vi "Comparison of Streaming File Formats.vi"() -> ()   [LabVIEW 2023]
doc: "The Comparison of Streaming File Formats example acquires images and then saves them to disk using a variety of file formats and options. Then it reads those images from disk and compares them with the original acquired images to report the file size, write time, and whether the saved image exactly matches the acquired image. \n\nIt's important to note this example only saves a few images and you may see different results when saving a larger number of images. You should also ensure the drive where the files are saved matches the desired location since different drives may have different performance. \n\nTo view an example of how to acquire images from a camera while saving to disk, see the Stream to Disk examples."
uses:
  <vilib>/Utility/miscctls.llb/LVRowAndColumnUnsignedTypeDef.ctl
  <vilib>/vision/Avi.llb/IMAQ AVI2 Codec Path.ctl
  <vilib>/Analysis/baseanly.llb/Mean (DBL).vi
  <vilib>/Utility/High Resolution Relative Seconds.vi
  SubVIs/TDMS File Initialization (Write).vi
  <vilib>/vision/EDVR.llb/IMAQ ImageToEDVR.vi
  <vilib>/vision/EDVR.llb/IMAQ ImageToEDVR 1D U8.vi
  <vilib>/vision/EDVR.llb/IMAQ ImageToEDVR 1D I16.vi
  <vilib>/vision/EDVR.llb/IMAQ ImageToEDVR 1D U32.vi
  <vilib>/vision/EDVR.llb/IMAQ ImageToEDVR 1D U16.vi
  SubVIs/TDMS File Initialization (Read).vi
  <vilib>/Analysis/NI_AALBase.lvlib
  <vilib>/vision/driver/NI_Vision_Acquisition_Software.lvlib
panel:
  out "TDMS Disable Buffering":bool
  in  "Number of Images to Save for Each File Format":u32=25
  in  "Show Only Lossless":bool=TRUE
  out "Destination Folder":path
  in  "Camera Name":refnum<k21> caption="IMAQdx Session"
  in  "Stop":bool
  in  "Sort By":enum16{"Write Time", "File Size"}(ring)
  out "Results":i32(listbox)=-1
  out "Progress Bar":i32(slide) max=39 scale=0.0..39.0
  # "Overview: Demonstrates how to save images to disk using a variety of file formats and then reads them back and compares file size, write time, and whether the saved image exactly maches the acquired image. \nRequirements: Vision Acquisition Software.\nInstructions:\n1. Select the Camera Name.\n2. Run the VI\n3. When the table is populated, use Show Only Lossless and Sort By to modify the displayed results."
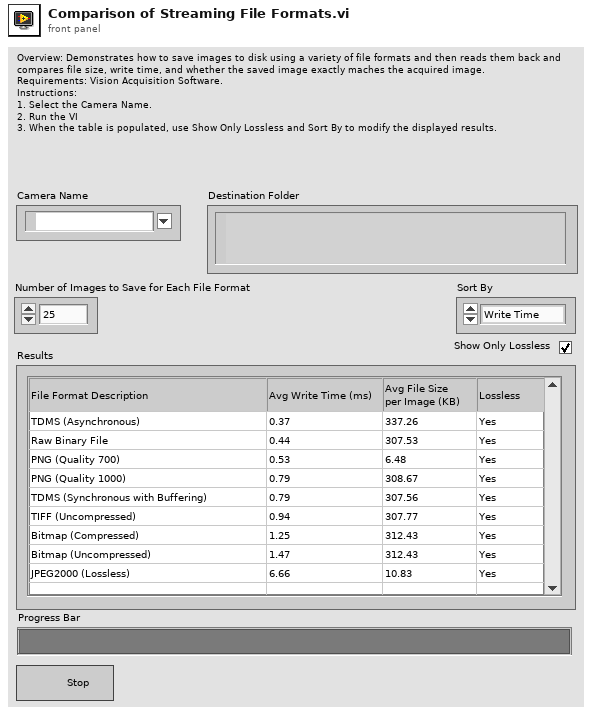
[diagram p1: front panel]
types:
  T1 = typedef "LVRowAndColumnUnsignedTypeDef.ctl" = cluster{"Row":u32, "Column":u32}
  T2 = enum8{"Enabled", "Disabled", "Disabled and Grayed Out"}
  T3 = typedef "IMAQ Image.ctl" = refnum<image>
  T4 = typedef "IMAQdx.ctl" = refnum<k21>
  T5 = typedef "Image Type" = u32
  T6 = cluster{"Rows Per Strip":i32, "Photometric":i32, "Compression Type":i32}
  T7 = cluster{"Asynchronous":bool, "Disable Buffering if Supported":bool, "Reserved Images":i64, "Fail if Reservation Fails":bool}
  T8 = enum16{"open", "replace", "create", "open or create", "replace or create", "replace or create with confirmation"}
  T9 = cluster{"Table Data":string[], "Description":string, "Write time":dbl, "File Size":dbl, "Sort Quality":dbl}
  T10 = typedef "IMAQ AVI2 Codec Path.ctl" = u32
  T11 = cluster{"Image Type":T5, "Async File Format":bool}
  T12 = cluster{"Asynchronous Write":bool, "Reserve Disk Space":bool, "Disable Buffering":bool}
  T13 = typedef "IMAQ AVI2 Refnum.ctl" = refnum<k20>
  T14 = typedef "TDMS Read Data.ctl" = cluster{"Image Type":T5, "Width":u32, "Height":u32, "Pixels per Image":u32, "Total Width":u32, "Left Offset":u32, "Image":T3}
  T15 = cluster{"Write time":dbl, "Sort Quality":dbl, "Table Data":string[]}
  T16 = cluster{"Write time":dbl, "Sort Quality":dbl, "Table Data":string[]}[]
  T17 = cluster{"File Size":dbl, "Sort Quality":dbl, "Table Data":string[]}
  T18 = cluster{"File Size":dbl, "Sort Quality":dbl, "Table Data":string[]}[]
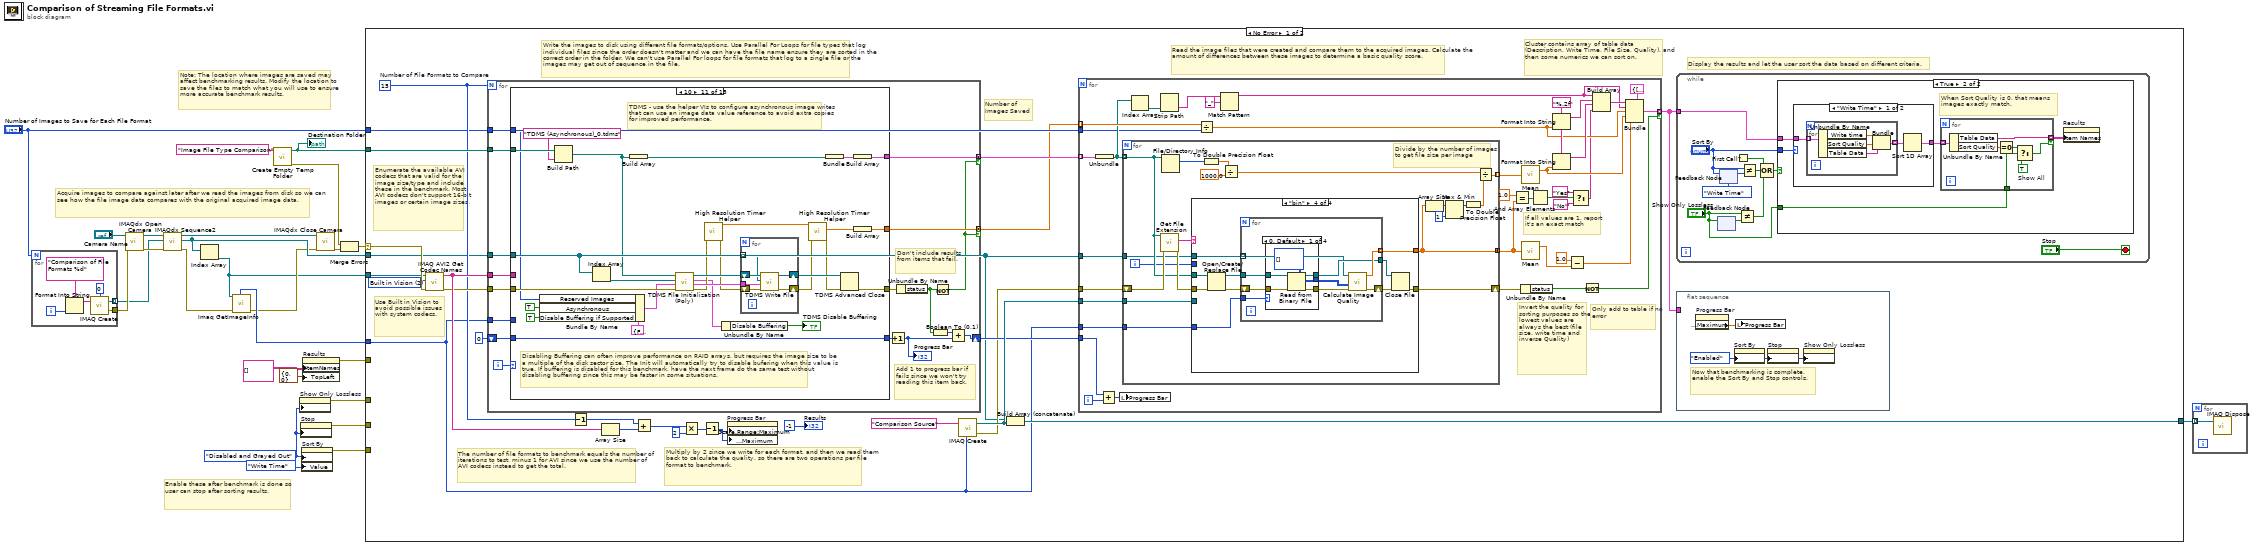
[diagram p0: block diagram]
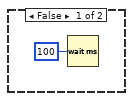
[diagram p2: hidden frame]
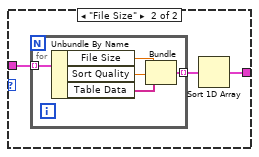
[diagram p3: hidden frame]
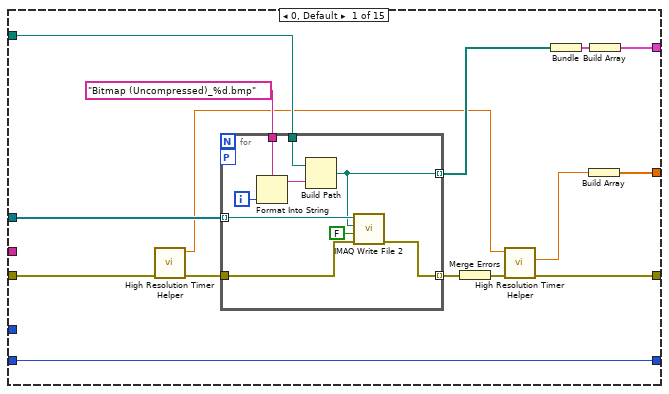
[diagram p4: hidden frame]
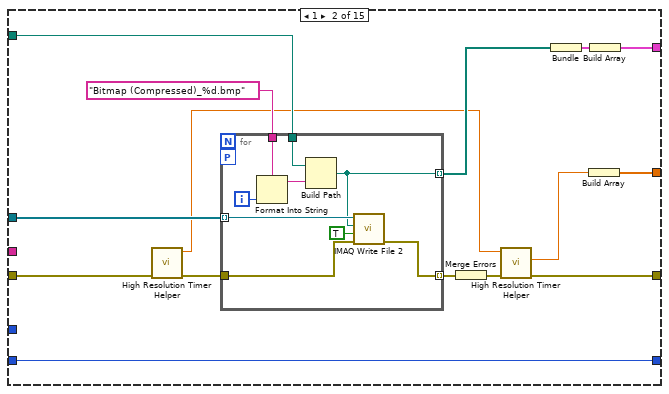
[diagram p5: hidden frame]
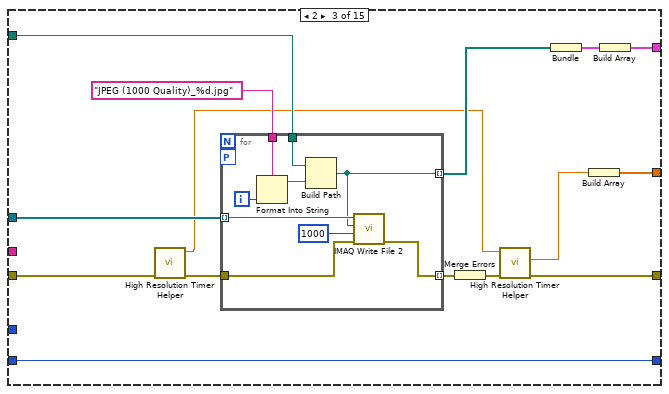
[diagram p6: hidden frame]
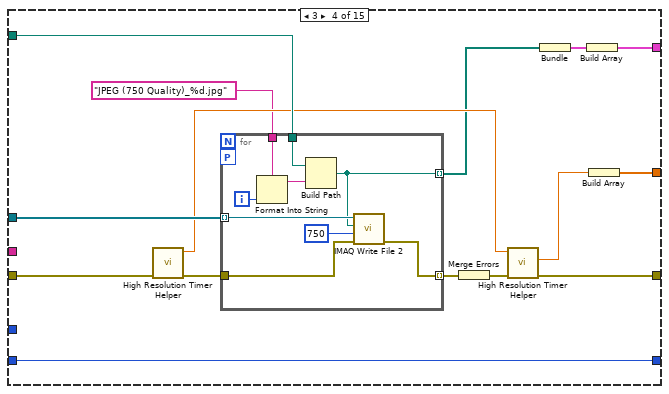
[diagram p7: hidden frame]
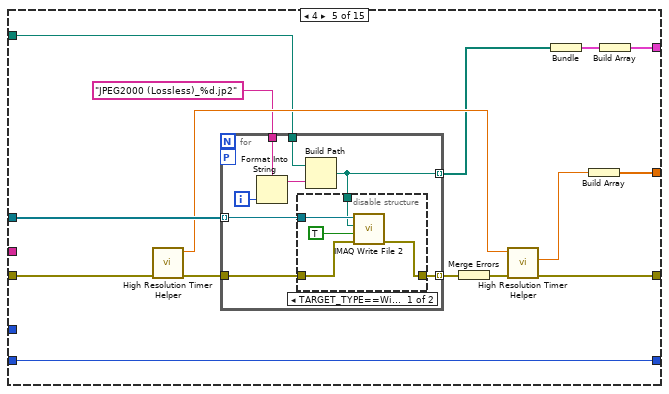
[diagram p8: hidden frame]
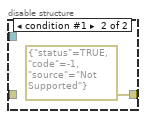
[diagram p9: hidden frame]
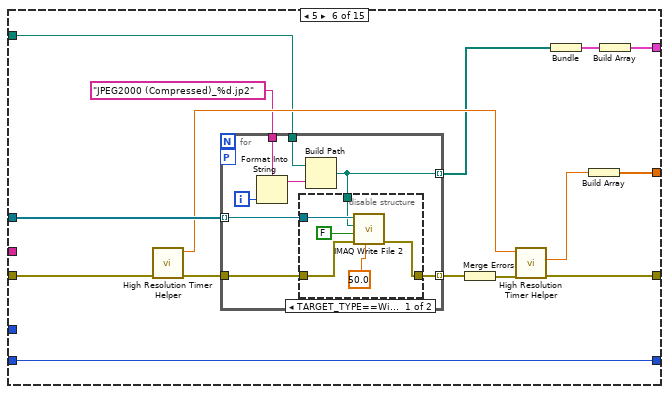
[diagram p10: hidden frame]
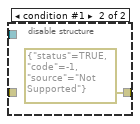
[diagram p11: hidden frame]
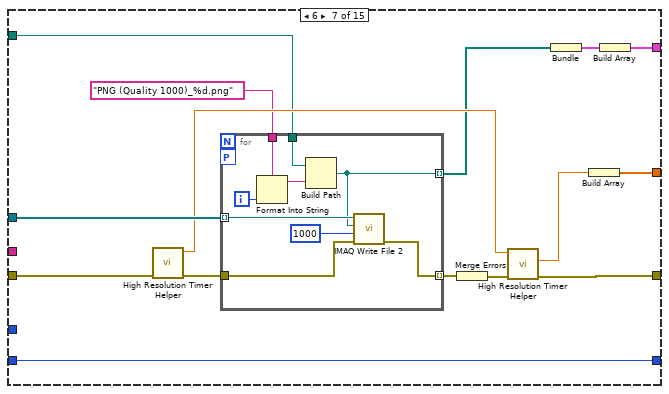
[diagram p12: hidden frame]
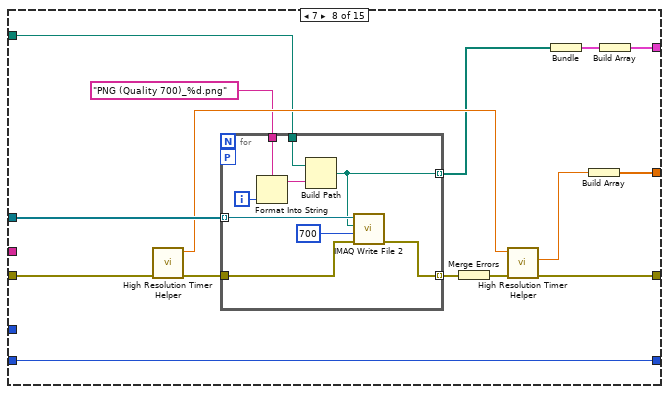
[diagram p13: hidden frame]
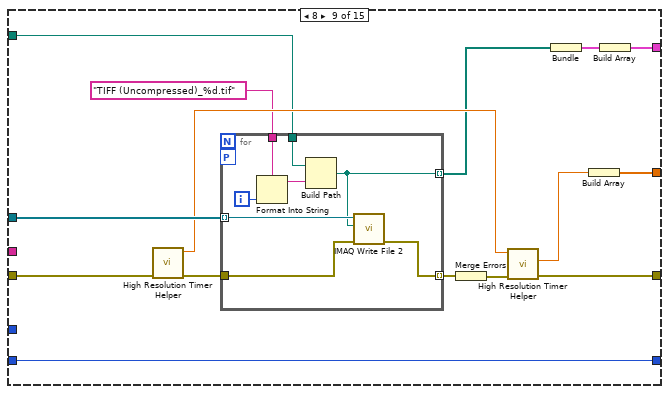
[diagram p14: hidden frame]
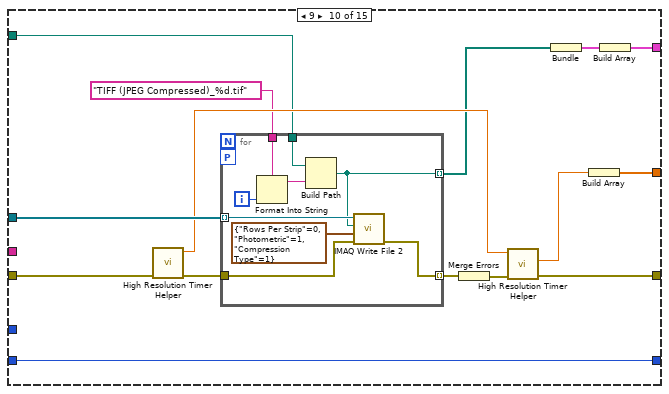
[diagram p15: hidden frame]
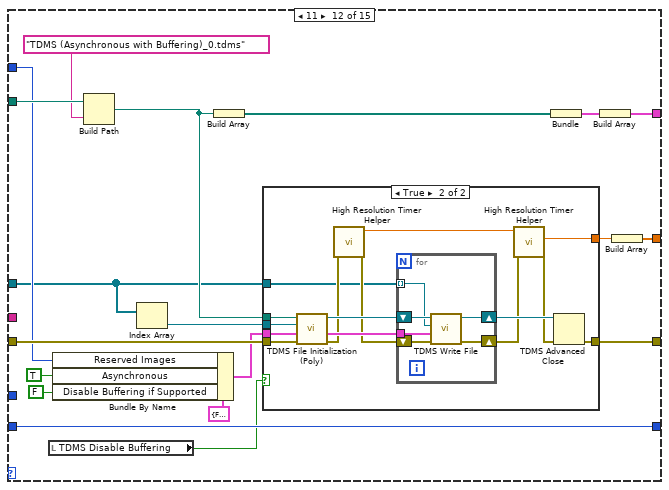
[diagram p16: hidden frame]
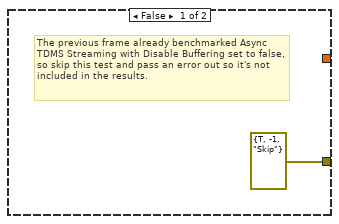
[diagram p17: hidden frame]
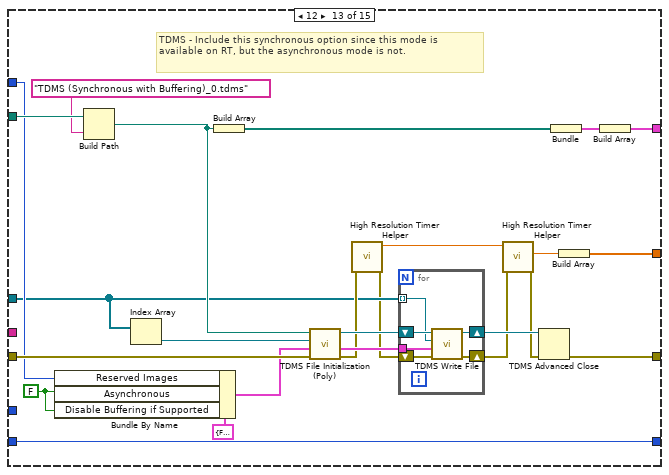
[diagram p18: hidden frame]
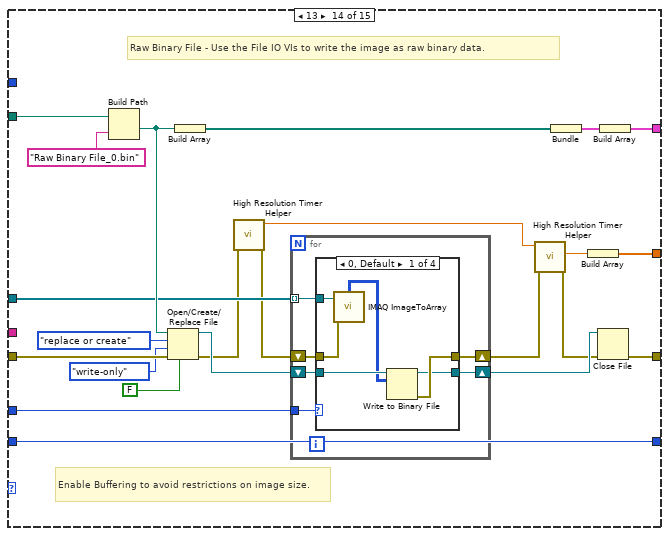
[diagram p19: hidden frame]
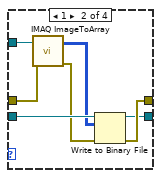
[diagram p20: hidden frame]
diagram:
  w16 = T2."Disabled and Grayed Out" ("Disabled")
  # "Note: The location where images are saved may affect benchmarking results. Modify the location to save the files to match what you will use to ensure more accurate benchmark results."
  # "Enable these after benchmark is done so user can stop after sorting results."
  # "Acquire images to compare against later after we read the images from disk so we can see how the file image data compares with the original acquired image data."
  n1 = for {
    N: "Number of Images to Save for Each File Format" -> [_]
    tunnel: [w32] -> w10
    tunnel: [w28] -> w1 mode=indexing
    i -> [w29]
    n2 = Format Into String(format string="Comparison of File Formats %d", w29) -> (resulting string=w30:string)  [unwired: 2 in, 1 out]
    n3 = call "IMAQ Create"("Border Size"=0, "Image Name"=w30) -> ("New Image"=w28:T3, "error out"=w32:errorcluster)  [unwired: 3 in]
  }
  n4 = call <vilib>:"IMAQdx Open Camera.vi"("error in"=w10, "Session In"="Camera Name") -> ("error out"=w8:errorcluster, "Session Out"=w9:T4)  [unwired: 8 in]
  n5 = call <vilib>:"IMAQdx Sequence2.vi"("error in"=w8, "Images In"=w1, "Session In"=w9) -> ("error out"=w7:errorcluster, "Images Out"=w5:T3[], "Session Out"=w6:T4)  [unwired: 6 in]
  n6 = Index Array(array=w5) -> (element=w2:T3)  [unwired: 1 in]
  n7 = call "Imaq GetImageInfo"("error in (no error)"=w7, "Image"=w2) -> ("error out"=w4:errorcluster, "Image Type"=w11:T5)  [unwired: 2 in, 6 out]
  n8 = call "Create Empty Temp Folder.vi"("Folder Name"="Image File Type Comparison") -> ("error out"=w12:errorcluster, "Empty Temp Folder"=w13:path)  [unwired: 9 in]
  "Destination Folder" <- w13
  n9 = property on="Show Only Lossless" class="Bool (strict)"("DisabledEnum"=w16) -> (error out=w15:errorcluster)  [unwired: 2 in, 1 out]
  n10 = property on="Stop" class="Bool"("DisabledEnum"=w16) -> (error out=w25:errorcluster)  [unwired: 2 in, 1 out]
  n11 = property on="Sort By" class="Enum (strict)"("DisabledEnum"=w16, "Value"=enum16{"Write Time", "File Size"}."Write Time" ("Sort By")) -> (error out=w24:errorcluster)  [unwired: 2 in, 1 out]
  n12 = property on="Results" class="MCListbox (strict)"("ItemNames"=string[][] [] ("Item Names"), "TopLeft"=T1 {"Row"=0, "Column"=0} ("Top Left Visible Cell")) -> (error out=w19:errorcluster)  [unwired: 2 in, 1 out]
  n13 = call <vilib>:"IMAQdx Close Camera.vi"("error in"=w4, "Session In"=w6) -> ("error out"=w22:errorcluster)  [unwired: 9 in]
  n14 = Merge Errors(w12, w22) -> (w21:errorcluster)
  n15 = case shown="No Error" w21 {
    selector: w21 -> [w42 w718]
    tunnel: [w54 w717] -> w26
    tunnel: w13 -> [w52 _]
    tunnel: w5 -> [w35 w717]
    tunnel: w25 -> [_ _]
    tunnel: w24 -> [_ _]
    tunnel: w19 -> [_ _]
    tunnel: w15 -> [_ _]
    tunnel: w11 -> [w38 _]
    tunnel: "Number of Images to Save for Each File Format" -> [w36 _]
    tunnel: w2 -> [w37 _]
    frame No Error {
      w34 = T10 2 items=["Default", "System", "Built in Vision"] ("Codec Source")
      w44 = 15  # Number of File Formats to Compare
      # "Use Built in Vision to avoid possible issues with system codecs."
      # "Number of Images Saved"
      # "Cluster contains array of table data (Description, Write Time, File Size, Quality), and then some numerics we can sort on."
      # "Display the results and let the user sort the data based on different criteria."
      # "The number of file formats to benchmark equals the number of iterations to test, minus 1 for AVI since we use the number of AVI codecs instead to get the total."
      # "Write the images to disk using different file formats/options. Use Parallel For Loops for file types that log individual files since the order doesn't matter and we can have the file name ensure they are sorted in the correct order in the folder. We can't use Parallel For loops for file formats that log to a single file or the images may get out of sequence in the file."
      # "Read the image files that were created and compare them to the acquired images. Calculate the amount of differences between these images to determine a basic quality score."
      # "Multiply by 2 since we write for each format, and then we read them back to calculate the quality, so there are two operations per file format to benchmark."
      # "Enumerate the available AVI codecs that are valid for the image size/type and include these in the benchmark. Most AVI codecs don't support 16-bit images or certain image sizes."
      n16 = call "IMAQ AVI2 Get Codec Names"("error in (no error)"=w42, "Codec Source"=w34, "Image"=w37) -> ("error out"=w48:errorcluster, "Codec Names"=w51:string[])  [unwired: 7 out]
      n17 = for {
        N: w44 -> [_]
        tunnel: [w117] -> w33 mode=concatenating if=w109
        tunnel: w52 -> [w116]
        tunnel: w51 -> [w115]
        tunnel: w48 -> [w114]
        tunnel: w35 -> [w113]
        tunnel: [w112] -> w46 mode=concatenating if=w109
        shift-right: [w106] -> w45
        shift-left: 0 -> [w111]
        tunnel: w38 -> [w110]
        tunnel: w36 -> [w101]
        i -> [w102]
        # "Add 1 to progress bar if fails since we won't try reading this item back."
        # "Don't include results from items that fail."
        n18 = case shown="10" w102 {
          tunnel: [w131 w155 w179 w202 w225 w254 w284 w308 w332 w355 w395 w420 w467 w496 w537] -> w117
          tunnel: [w120 w144 w168 w198 w218 w247 w277 w301 w325 w348 w386 w411 w460 w484 w536] -> w103
          tunnel: w116 -> [w130 w154 w178 w201 w224 w253 w283 w307 w331 w354 w390 w415 w463 w492 w535]
          tunnel: w115 -> [_ _ _ _ _ _ _ _ _ _ _ _ _ _ w534]
          tunnel: w114 -> [w123 w147 w171 w203 w226 w255 w285 w309 w333 w356 w391 w416 w456 w488 w533]
          tunnel: w113 -> [w132 w156 w180 w204 w228 w257 w287 w311 w335 w358 w370 w403 w445 w480 w531]
          tunnel: [w129 w153 w177 w200 w220 w249 w279 w303 w327 w350 w393 w418 w465 w494 w532] -> w112
          tunnel: w111 -> [w125 w149 w176 w199 w219 w248 w278 w302 w326 w349 w392 w417 w464 w493 w530]
          tunnel: [w125 w149 w176 w199 w219 w248 w278 w302 w326 w349 w392 w417 w464 w493 w529] -> w105
          tunnel: w110 -> [_ _ _ _ _ _ _ _ _ _ _ _ _ w489 _]
          tunnel: w101 -> [_ _ _ _ _ _ _ _ _ _ w368 w404 w446 _ _]
          frame 0, Default {
            n19 = call "High Resolution Timer Helper.vi"("error in (no error)"=w123) -> ("error out"=w122:errorcluster, "Current Time"=w119:dbl)  [unwired: 8 in, 1 out]
            n20 = for {
              tunnel: w132 -> [w141] mode=indexing
              tunnel: w130 -> [w139]
              tunnel: "Bitmap (Uncompressed)_%d.bmp" -> [w137]
              tunnel: [w135] -> w127 mode=indexing
              workers-P: _ -> [_]
              tunnel: w122 -> [w134]
              tunnel: [w133] -> w124 mode=indexing
              i -> [w138]
              n21 = Format Into String(format string=w137, w138) -> (resulting string=w136:string)  [unwired: 2 in, 1 out]
              n22 = Build Path(base path=w139, name or relative path=w136) -> (appended path=w135:path)
              n23 = call-poly "IMAQ Write File 2"("error in (no error)"=w134, "Compress? (N)"=FALSE, "File Path"=w135, "Image"=w141) -> ("error out"=w133:errorcluster)  [unwired: 6 in, 1 out]
            }
            n24 = Merge Errors(w124) -> (w121:errorcluster)
            n25 = call "High Resolution Timer Helper.vi"("error in (no error)"=w121, "Previous Time"=w119) -> ("error out"=w120:errorcluster, "Time Difference (ms)"=w118:dbl)  [unwired: 7 in, 1 out]
            n26 = Bundle(w127) -> (w126:cluster{path[]})  [unwired: 1 in]
            n27 = Build Array(w118) -> (w131:dbl[])
            n28 = Build Array(w126) -> (w129:cluster{path[]}[])
          }
          frame 1 {
            n29 = call "High Resolution Timer Helper.vi"("error in (no error)"=w147) -> ("error out"=w146:errorcluster, "Current Time"=w142:dbl)  [unwired: 8 in, 1 out]
            n30 = for {
              tunnel: w156 -> [w165] mode=indexing
              tunnel: w154 -> [w163]
              tunnel: "Bitmap (Compressed)_%d.bmp" -> [w161]
              tunnel: [w159] -> w151 mode=indexing
              workers-P: _ -> [_]
              tunnel: w146 -> [w158]
              tunnel: [w157] -> w148 mode=indexing
              i -> [w162]
              n31 = Format Into String(format string=w161, w162) -> (resulting string=w160:string)  [unwired: 2 in, 1 out]
              n32 = Build Path(base path=w163, name or relative path=w160) -> (appended path=w159:path)
              n33 = call-poly "IMAQ Write File 2"("error in (no error)"=w158, "Compress? (N)"=TRUE, "File Path"=w159, "Image"=w165) -> ("error out"=w157:errorcluster)  [unwired: 6 in, 1 out]
            }
            n34 = Merge Errors(w148) -> (w145:errorcluster)
            n35 = call "High Resolution Timer Helper.vi"("error in (no error)"=w145, "Previous Time"=w142) -> ("error out"=w144:errorcluster, "Time Difference (ms)"=w143:dbl)  [unwired: 7 in, 1 out]
            n36 = Bundle(w151) -> (w150:cluster{path[]})  [unwired: 1 in]
            n37 = Build Array(w143) -> (w155:dbl[])
            n38 = Build Array(w150) -> (w153:cluster{path[]}[])
          }
          frame 2 {
            n39 = call "High Resolution Timer Helper.vi"("error in (no error)"=w171) -> ("error out"=w170:errorcluster, "Current Time"=w166:dbl)  [unwired: 8 in, 1 out]
            n40 = for {
              tunnel: w180 -> [w189] mode=indexing
              tunnel: w178 -> [w188]
              tunnel: "JPEG (1000 Quality)_%d.jpg" -> [w186]
              tunnel: [w184] -> w174 mode=indexing
              workers-P: _ -> [_]
              tunnel: w170 -> [w182]
              tunnel: [w181] -> w172 mode=indexing
              i -> [w187]
              n41 = Format Into String(format string=w186, w187) -> (resulting string=w185:string)  [unwired: 2 in, 1 out]
              n42 = Build Path(base path=w188, name or relative path=w185) -> (appended path=w184:path)
              n43 = call-poly "IMAQ Write File 2"("error in (no error)"=w182, "Image Quality"=u32 1000, "File Path"=w184, "Image"=w189) -> ("error out"=w181:errorcluster)  [unwired: 6 in, 1 out]
            }
            n44 = Merge Errors(w172) -> (w169:errorcluster)
            n45 = call "High Resolution Timer Helper.vi"("error in (no error)"=w169, "Previous Time"=w166) -> ("error out"=w168:errorcluster, "Time Difference (ms)"=w167:dbl)  [unwired: 7 in, 1 out]
            n46 = Bundle(w174) -> (w173:cluster{path[]})  [unwired: 1 in]
            n47 = Build Array(w167) -> (w179:dbl[])
            n48 = Build Array(w173) -> (w177:cluster{path[]}[])
          }
          frame 3 {
            n49 = call "High Resolution Timer Helper.vi"("error in (no error)"=w203) -> ("error out"=w192:errorcluster, "Current Time"=w197:dbl)  [unwired: 8 in, 1 out]
            n50 = for {
              tunnel: w204 -> [w213] mode=indexing
              tunnel: w201 -> [w212]
              tunnel: "JPEG (750 Quality)_%d.jpg" -> [w210]
              tunnel: [w208] -> w195 mode=indexing
              workers-P: _ -> [_]
              tunnel: w192 -> [w206]
              tunnel: [w205] -> w191 mode=indexing
              i -> [w211]
              n51 = Format Into String(format string=w210, w211) -> (resulting string=w209:string)  [unwired: 2 in, 1 out]
              n52 = Build Path(base path=w212, name or relative path=w209) -> (appended path=w208:path)
              n53 = call-poly "IMAQ Write File 2"("error in (no error)"=w206, "Image Quality"=u32 750, "File Path"=w208, "Image"=w213) -> ("error out"=w205:errorcluster)  [unwired: 6 in, 1 out]
            }
            n54 = Merge Errors(w191) -> (w190:errorcluster)
            n55 = call "High Resolution Timer Helper.vi"("error in (no error)"=w190, "Previous Time"=w197) -> ("error out"=w198:errorcluster, "Time Difference (ms)"=w193:dbl)  [unwired: 7 in, 1 out]
            n56 = Bundle(w195) -> (w194:cluster{path[]})  [unwired: 1 in]
            n57 = Build Array(w194) -> (w200:cluster{path[]}[])
            n58 = Build Array(w193) -> (w202:dbl[])
          }
          frame 4 {
            n59 = call "High Resolution Timer Helper.vi"("error in (no error)"=w226) -> ("error out"=w216:errorcluster, "Current Time"=w227:dbl)  [unwired: 8 in, 1 out]
            n60 = for {
              tunnel: w228 -> [w236] mode=indexing
              tunnel: w224 -> [w235]
              tunnel: "JPEG2000 (Lossless)_%d.jp2" -> [w233]
              tunnel: [w231] -> w222 mode=indexing
              workers-P: _ -> [_]
              tunnel: w216 -> [w230]
              tunnel: [w229] -> w215 mode=indexing
              i -> [w234]
              n61 = Format Into String(format string=w233, w234) -> (resulting string=w232:string)  [unwired: 2 in, 1 out]
              n62 = Build Path(base path=w235, name or relative path=w232) -> (appended path=w231:path)
              n63 = disable-structure shown="TARGET_TYPE==Windows" {
                disable-tunnel: w236 -> [w241 _]
                disable-tunnel: w230 -> [w240 _]
                disable-tunnel: [w239 errorcluster {"status"=TRUE, "code"=-1, "source"="Not Supported"} ("error out")] -> w229
                disable-tunnel: w231 -> [w238 _]
                frame condition #0 (active) {
                  n64 = call-poly "IMAQ Write File 2"("error in (no error)"=w240, "Lossless? (true)"=TRUE, "File Path"=w238, "Image"=w241) -> ("error out"=w239:errorcluster)  [unwired: 6 in, 1 out]
                }
                frame condition #1 {
                }
              }
            }
            n65 = Merge Errors(w215) -> (w214:errorcluster)
            n66 = call "High Resolution Timer Helper.vi"("error in (no error)"=w214, "Previous Time"=w227) -> ("error out"=w218:errorcluster, "Time Difference (ms)"=w217:dbl)  [unwired: 7 in, 1 out]
            n67 = Bundle(w222) -> (w221:cluster{path[]})  [unwired: 1 in]
            n68 = Build Array(w217) -> (w225:dbl[])
            n69 = Build Array(w221) -> (w220:cluster{path[]}[])
          }
          frame 5 {
            n70 = call "High Resolution Timer Helper.vi"("error in (no error)"=w255) -> ("error out"=w245:errorcluster, "Current Time"=w256:dbl)  [unwired: 8 in, 1 out]
            n71 = for {
              tunnel: w257 -> [w265] mode=indexing
              tunnel: w253 -> [w264]
              tunnel: "JPEG2000 (Compressed)_%d.jp2" -> [w262]
              tunnel: [w260] -> w251 mode=indexing
              workers-P: _ -> [_]
              tunnel: w245 -> [w259]
              tunnel: [w258] -> w244 mode=indexing
              i -> [w263]
              n72 = Format Into String(format string=w262, w263) -> (resulting string=w261:string)  [unwired: 2 in, 1 out]
              n73 = Build Path(base path=w264, name or relative path=w261) -> (appended path=w260:path)
              n74 = disable-structure shown="TARGET_TYPE==Windows" {
                disable-tunnel: w265 -> [w271 _]
                disable-tunnel: w259 -> [w270 _]
                disable-tunnel: [w269 errorcluster {"status"=TRUE, "code"=-1, "source"="Not Supported"} ("error out")] -> w258
                disable-tunnel: w260 -> [w268 _]
                frame condition #0 (active) {
                  n75 = call-poly "IMAQ Write File 2"("Compression Ratio"=sgl 50.0, "error in (no error)"=w270, "Lossless? (true)"=FALSE, "File Path"=w268, "Image"=w271) -> ("error out"=w269:errorcluster)  [unwired: 5 in, 1 out]
                }
                frame condition #1 {
                }
              }
            }
            n76 = Merge Errors(w244) -> (w243:errorcluster)
            n77 = call "High Resolution Timer Helper.vi"("error in (no error)"=w243, "Previous Time"=w256) -> ("error out"=w247:errorcluster, "Time Difference (ms)"=w246:dbl)  [unwired: 7 in, 1 out]
            n78 = Bundle(w251) -> (w250:cluster{path[]})  [unwired: 1 in]
            n79 = Build Array(w246) -> (w254:dbl[])
            n80 = Build Array(w250) -> (w249:cluster{path[]}[])
          }
          frame 6 {
            n81 = call "High Resolution Timer Helper.vi"("error in (no error)"=w285) -> ("error out"=w275:errorcluster, "Current Time"=w286:dbl)  [unwired: 8 in, 1 out]
            n82 = for {
              tunnel: w287 -> [w296] mode=indexing
              tunnel: w283 -> [w295]
              tunnel: "PNG (Quality 1000)_%d.png" -> [w293]
              tunnel: [w291] -> w281 mode=indexing
              workers-P: _ -> [_]
              tunnel: w275 -> [w289]
              tunnel: [w288] -> w274 mode=indexing
              i -> [w294]
              n83 = Format Into String(format string=w293, w294) -> (resulting string=w292:string)  [unwired: 2 in, 1 out]
              n84 = Build Path(base path=w295, name or relative path=w292) -> (appended path=w291:path)
              n85 = call-poly "IMAQ Write File 2"("error in (no error)"=w289, "Image Quality"=u32 1000, "File Path"=w291, "Image"=w296) -> ("error out"=w288:errorcluster)  [unwired: 6 in, 1 out]
            }
            n86 = Merge Errors(w274) -> (w273:errorcluster)
            n87 = call "High Resolution Timer Helper.vi"("error in (no error)"=w273, "Previous Time"=w286) -> ("error out"=w277:errorcluster, "Time Difference (ms)"=w276:dbl)  [unwired: 7 in, 1 out]
            n88 = Bundle(w281) -> (w280:cluster{path[]})  [unwired: 1 in]
            n89 = Build Array(w276) -> (w284:dbl[])
            n90 = Build Array(w280) -> (w279:cluster{path[]}[])
          }
          frame 7 {
            n91 = call "High Resolution Timer Helper.vi"("error in (no error)"=w309) -> ("error out"=w299:errorcluster, "Current Time"=w310:dbl)  [unwired: 8 in, 1 out]
            n92 = for {
              tunnel: w311 -> [w320] mode=indexing
              tunnel: w307 -> [w319]
              tunnel: "PNG (Quality 700)_%d.png" -> [w317]
              tunnel: [w315] -> w305 mode=indexing
              workers-P: _ -> [_]
              tunnel: w299 -> [w313]
              tunnel: [w312] -> w298 mode=indexing
              i -> [w318]
              n93 = Format Into String(format string=w317, w318) -> (resulting string=w316:string)  [unwired: 2 in, 1 out]
              n94 = Build Path(base path=w319, name or relative path=w316) -> (appended path=w315:path)
              n95 = call-poly "IMAQ Write File 2"("error in (no error)"=w313, "Image Quality"=u32 700, "File Path"=w315, "Image"=w320) -> ("error out"=w312:errorcluster)  [unwired: 6 in, 1 out]
            }
            n96 = Merge Errors(w298) -> (w297:errorcluster)
            n97 = call "High Resolution Timer Helper.vi"("error in (no error)"=w297, "Previous Time"=w310) -> ("error out"=w301:errorcluster, "Time Difference (ms)"=w300:dbl)  [unwired: 7 in, 1 out]
            n98 = Bundle(w305) -> (w304:cluster{path[]})  [unwired: 1 in]
            n99 = Build Array(w300) -> (w308:dbl[])
            n100 = Build Array(w304) -> (w303:cluster{path[]}[])
          }
          frame 8 {
            n101 = call "High Resolution Timer Helper.vi"("error in (no error)"=w333) -> ("error out"=w323:errorcluster, "Current Time"=w334:dbl)  [unwired: 8 in, 1 out]
            n102 = for {
              tunnel: w335 -> [w343] mode=indexing
              tunnel: w331 -> [w342]
              tunnel: "TIFF (Uncompressed)_%d.tif" -> [w340]
              tunnel: [w338] -> w329 mode=indexing
              workers-P: _ -> [_]
              tunnel: w323 -> [w337]
              tunnel: [w336] -> w322 mode=indexing
              i -> [w341]
              n103 = Format Into String(format string=w340, w341) -> (resulting string=w339:string)  [unwired: 2 in, 1 out]
              n104 = Build Path(base path=w342, name or relative path=w339) -> (appended path=w338:path)
              n105 = call-poly "IMAQ Write File 2"("error in (no error)"=w337, "File Path"=w338, "Image"=w343) -> ("error out"=w336:errorcluster)  [unwired: 7 in, 1 out]
            }
            n106 = Merge Errors(w322) -> (w321:errorcluster)
            n107 = call "High Resolution Timer Helper.vi"("error in (no error)"=w321, "Previous Time"=w334) -> ("error out"=w325:errorcluster, "Time Difference (ms)"=w324:dbl)  [unwired: 7 in, 1 out]
            n108 = Bundle(w329) -> (w328:cluster{path[]})  [unwired: 1 in]
            n109 = Build Array(w324) -> (w332:dbl[])
            n110 = Build Array(w328) -> (w327:cluster{path[]}[])
          }
          frame 9 {
            n111 = call "High Resolution Timer Helper.vi"("error in (no error)"=w356) -> ("error out"=w346:errorcluster, "Current Time"=w357:dbl)  [unwired: 8 in, 1 out]
            n112 = for {
              tunnel: w358 -> [w367] mode=indexing
              tunnel: w354 -> [w366]
              tunnel: "TIFF (JPEG Compressed)_%d.tif" -> [w364]
              tunnel: [w362] -> w352 mode=indexing
              workers-P: _ -> [_]
              tunnel: w346 -> [w360]
              tunnel: [w359] -> w345 mode=indexing
              i -> [w365]
              n113 = Format Into String(format string=w364, w365) -> (resulting string=w363:string)  [unwired: 2 in, 1 out]
              n114 = Build Path(base path=w366, name or relative path=w363) -> (appended path=w362:path)
              n115 = call-poly "IMAQ Write File 2"("error in (no error)"=w360, "TIFF Options"=T6 {"Rows Per Strip"=0, "Photometric"=1, "Compression Type"=1}, "File Path"=w362, "Image"=w367) -> ("error out"=w359:errorcluster)  [unwired: 6 in, 1 out]
            }
            n116 = Merge Errors(w345) -> (w344:errorcluster)
            n117 = call "High Resolution Timer Helper.vi"("error in (no error)"=w344, "Previous Time"=w357) -> ("error out"=w348:errorcluster, "Time Difference (ms)"=w347:dbl)  [unwired: 7 in, 1 out]
            n118 = Bundle(w352) -> (w351:cluster{path[]})  [unwired: 1 in]
            n119 = Build Array(w347) -> (w355:dbl[])
            n120 = Build Array(w351) -> (w350:cluster{path[]}[])
          }
          frame 10 {
            # "Disabling Buffering can often improve performance on RAID arrays, but requires the image size to be a multiple of the disk sector size. The Init will automatically try to disable bufering when this value is true. If buffering is disabled for this benchmark, have the next frame do the same test without disabling buffering since this may be faster in some situations."
            # "TDMS - use the helper VIs to configure asynchronous image writes that can use an image data value reference to avoid extra copies for improved performance."
            n121 = Bundle By Name(cluster=T7 {"Asynchronous"=FALSE, "Disable Buffering if Supported"=FALSE, "Reserved Images"=1000, "Fail if Reservation Fails"=FALSE} ("Write Settings"), "Reserved Images"=w368, "Asynchronous"=TRUE, "Disable Buffering if Supported"=TRUE ("Asynchronous")) -> (w372:T7)
            n122 = Build Path(base path=w390, name or relative path="TDMS (Asynchronous)_0.tdms") -> (appended path=w388:path)
            n123 = Index Array(array=w370) -> (element=w369:T3)  [unwired: 1 in]
            n124 = Build Array(w388) -> (w387:path[])
            n125 = call-poly "TDMS File Initialization (Poly).vi"("error in (no error)"=w391, "Write Settings"=w372, "Image In"=w369, "File Path"=w388) -> ("error out"=w382:errorcluster, "Write Settings Out"=w383:T11, "Optimizations Configured"=w376:T12, "TDMS Refnum Out"=w384:refnum<k34>)  [unwired: 4 in]
            n126 = call "High Resolution Timer Helper.vi"("error in (no error)"=w382) -> ("error out"=w381:errorcluster, "Current Time"=w378:dbl)  [unwired: 8 in, 1 out]
            n127 = Unbundle By Name(w376) -> ("Disable Buffering"=→"TDMS Disable Buffering":bool)
            n128 = for {
              tunnel: w370 -> [w398] mode=indexing
              shift-right: [w396] -> w380
              shift-left: w381 -> [w401]
              shift-right: [w397] -> w385
              shift-left: w384 -> [w400]
              tunnel: w383 -> [w399]
              n129 = call "TDMS Write File.vi"("error in"=w401, "Write Settings"=w399, "Image"=w398, "TDMS Ref In"=w400) -> ("error out"=w396:errorcluster, "TDMS Ref Out"=w397:refnum<k34>)  [unwired: 6 in]
            }
            n130 = call "High Resolution Timer Helper.vi"("error in (no error)"=w380, "Previous Time"=w378) -> ("error out"=w379:errorcluster, "Time Difference (ms)"=w377:dbl)  [unwired: 7 in, 1 out]
            n131 = Bundle(w387) -> (w394:cluster{path[]})  [unwired: 1 in]
            n132 = TDMS Advanced Close(8:w379, 11:w385) -> (0:w386:errorcluster)  [unwired: 2 in, 1 out]
            n133 = Build Array(w394) -> (w393:cluster{path[]}[])
            n134 = Build Array(w377) -> (w395:dbl[])
          }
          frame 11 {
            n135 = local read "TDMS Disable Buffering"() -> (w406:bool)
            n136 = Bundle By Name(cluster=T7 {"Asynchronous"=FALSE, "Disable Buffering if Supported"=FALSE, "Reserved Images"=1000, "Fail if Reservation Fails"=FALSE} ("Write Settings"), "Reserved Images"=w404, "Asynchronous"=TRUE, "Disable Buffering if Supported"=FALSE) -> (w409:T7)
            n137 = Build Path(base path=w415, name or relative path="TDMS (Asynchronous with Buffering)_0.tdms") -> (appended path=w413:path)
            n138 = Index Array(array=w403) -> (element=w402:T3)  [unwired: 1 in]
            n139 = Build Array(w413) -> (w412:path[])
            n140 = case shown="True" w406 {
              tunnel: w416 -> [_ w436]
              tunnel: w413 -> [_ w435]
              tunnel: [errorcluster {"status"=TRUE, "code"=-1, "source"="Skip"} ("error out") w434] -> w411
              tunnel: [_ w425] -> w410
              tunnel: w403 -> [_ w424]
              tunnel: w409 -> [_ w423]
              tunnel: w402 -> [_ w422]
              frame False {
                # "The previous frame already benchmarked Async TDMS Streaming with Disable Buffering set to false, so skip this test and pass an error out so it's not included in the results."
              }
              frame True {
                n141 = call-poly "TDMS File Initialization (Poly).vi"("error in (no error)"=w436, "Write Settings"=w423, "Image In"=w422, "File Path"=w435) -> ("error out"=w430:errorcluster, "Write Settings Out"=w431:T11, "TDMS Refnum Out"=w432:refnum<k34>)  [unwired: 4 in, 1 out]
                n142 = call "High Resolution Timer Helper.vi"("error in (no error)"=w430) -> ("error out"=w429:errorcluster, "Current Time"=w426:dbl)  [unwired: 8 in, 1 out]
                n143 = for {
                  tunnel: w424 -> [w439] mode=indexing
                  shift-right: [w437] -> w428
                  shift-left: w429 -> [w442]
                  shift-right: [w438] -> w433
                  shift-left: w432 -> [w441]
                  tunnel: w431 -> [w440]
                  n144 = call "TDMS Write File.vi"("error in"=w442, "Write Settings"=w440, "Image"=w439, "TDMS Ref In"=w441) -> ("error out"=w437:errorcluster, "TDMS Ref Out"=w438:refnum<k34>)  [unwired: 6 in]
                }
                n145 = call "High Resolution Timer Helper.vi"("error in (no error)"=w428, "Previous Time"=w426) -> ("error out"=w427:errorcluster, "Time Difference (ms)"=w425:dbl)  [unwired: 7 in, 1 out]
                n146 = TDMS Advanced Close(8:w427, 11:w433) -> (0:w434:errorcluster)  [unwired: 2 in, 1 out]
              }
            }
            n147 = Bundle(w412) -> (w419:cluster{path[]})  [unwired: 1 in]
            n148 = Build Array(w419) -> (w418:cluster{path[]}[])
            n149 = Build Array(w410) -> (w420:dbl[])
          }
          frame 12 {
            w447 = FALSE ("Asynchronous")
            # "TDMS - Include this synchronous option since this mode is available on RT, but the asynchronous mode is not."
            n150 = Bundle By Name(cluster=T7 {"Asynchronous"=FALSE, "Disable Buffering if Supported"=FALSE, "Reserved Images"=1000, "Fail if Reservation Fails"=FALSE} ("Write Settings"), "Reserved Images"=w446, "Asynchronous"=w447, "Disable Buffering if Supported"=w447) -> (w455:T7)
            n151 = Build Path(base path=w463, name or relative path="TDMS (Synchronous with Buffering)_0.tdms") -> (appended path=w458:path)
            n152 = Index Array(array=w445) -> (element=w444:T3)  [unwired: 1 in]
            n153 = Build Array(w458) -> (w461:path[])
            n154 = call-poly "TDMS File Initialization (Poly).vi"("error in (no error)"=w456, "Write Settings"=w455, "Image In"=w444, "File Path"=w458) -> ("error out"=w453:errorcluster, "Write Settings Out"=w454:T11, "TDMS Refnum Out"=w457:refnum<k34>)  [unwired: 4 in, 1 out]
            n155 = call "High Resolution Timer Helper.vi"("error in (no error)"=w453) -> ("error out"=w443:errorcluster, "Current Time"=w451:dbl)  [unwired: 8 in, 1 out]
            n156 = for {
              tunnel: w445 -> [w471] mode=indexing
              shift-right: [w469] -> w450
              shift-left: w443 -> [w473]
              shift-right: [w468] -> w459
              shift-left: w457 -> [w472]
              tunnel: w454 -> [w470]
              n157 = call "TDMS Write File.vi"("error in"=w473, "Write Settings"=w470, "Image"=w471, "TDMS Ref In"=w472) -> ("error out"=w469:errorcluster, "TDMS Ref Out"=w468:refnum<k34>)  [unwired: 6 in]
            }
            n158 = call "High Resolution Timer Helper.vi"("error in (no error)"=w450, "Previous Time"=w451) -> ("error out"=w449:errorcluster, "Time Difference (ms)"=w452:dbl)  [unwired: 7 in, 1 out]
            n159 = TDMS Advanced Close(8:w449, 11:w459) -> (0:w460:errorcluster)  [unwired: 2 in, 1 out]
            n160 = Bundle(w461) -> (w466:cluster{path[]})  [unwired: 1 in]
            n161 = Build Array(w452) -> (w467:dbl[])
            n162 = Build Array(w466) -> (w465:cluster{path[]}[])
          }
          frame 13 {
            # "Raw Binary File - Use the File IO VIs to write the image as raw binary data."
            # "Enable Buffering to avoid restrictions on image size."
            n163 = Build Path(base path=w492, name or relative path="Raw Binary File_0.bin") -> (appended path=w487:path)
            n164 = Open/Create/Replace File(file path (use dialog)=w487, error in=w488, operation (0:open)=T8."replace or create", access (0:read/write)=enum16{"read/write", "read-only", "write-only"}."write-only", disable buffering (F)=FALSE) -> (refnum out=w485:refnum<file>, error out=w479:errorcluster)  [unwired: 1 in, 1 out]
            n165 = Build Array(w487) -> (w490:path[])
            n166 = call "High Resolution Timer Helper.vi"("error in (no error)"=w479) -> ("error out"=w474:errorcluster, "Current Time"=w477:dbl)  [unwired: 8 in, 1 out]
            n167 = for {
              shift-right: [w497] -> w476
              shift-left: w474 -> [w502]
              tunnel: w489 -> [w500]
              shift-right: [w499] -> w483
              shift-left: w485 -> [w501]
              tunnel: w480 -> [w498] mode=indexing
              n168 = case shown="0, Default" w500 {
                tunnel: w502 -> [w503 w512 w518 w524]
                tunnel: w501 -> [w508 w515 w522 w528]
                tunnel: [w507 w514 w521 w527] -> w497
                tunnel: [w506 w513 w520 w526] -> w499
                tunnel: w498 -> [w505 w511 w519 w525]
                frame 0, Default {
                  n169 = call "IMAQ ImageToArray"("error in (no error)"=w503, "Image"=w505) -> ("Image Pixels (U8)"=w504:u8[][])  [unwired: 2 in, 4 out]
                  n170 = Write to Binary File(file (use dialog)=w508, data=w504) -> (refnum out=w506:refnum<file>, error out=w507:errorcluster)  [unwired: 4 in, 1 out]
                }
                frame 1 {
                  n171 = call "IMAQ ImageToArray"("error in (no error)"=w512, "Image"=w511) -> ("error out"=w509:errorcluster, "Image Pixels (I16)"=w510:i16[][])  [unwired: 2 in, 3 out]
                  n172 = Write to Binary File(file (use dialog)=w515, data=w510, error in=w509) -> (refnum out=w513:refnum<file>, error out=w514:errorcluster)  [unwired: 3 in, 1 out]
                }
                frame 4 {
                  n173 = call "IMAQ ColorImageToArray"("Image"=w519, "error in (no error)"=w518) -> ("Image Pixels (U32)"=w517:u32[][], "error out"=w516:errorcluster)  [unwired: 2 in, 1 out]
                  n174 = Write to Binary File(file (use dialog)=w522, data=w517, error in=w516) -> (refnum out=w520:refnum<file>, error out=w521:errorcluster)  [unwired: 3 in, 1 out]
                }
                frame 7 {
                  n175 = call "IMAQ ImageToArray"("error in (no error)"=w524, "Image"=w525) -> ("Image Pixels (U16)"=w523:u16[][])  [unwired: 2 in, 4 out]
                  n176 = Write to Binary File(file (use dialog)=w528, data=w523) -> (refnum out=w526:refnum<file>, error out=w527:errorcluster)  [unwired: 4 in, 1 out]
                }
              }
            }
            n177 = call "High Resolution Timer Helper.vi"("error in (no error)"=w476, "Previous Time"=w477) -> ("error out"=w475:errorcluster, "Time Difference (ms)"=w478:dbl)  [unwired: 7 in, 1 out]
            n178 = Bundle(w490) -> (w495:cluster{path[]})  [unwired: 1 in]
            n179 = Build Array(w478) -> (w496:dbl[])
            n180 = Close File(refnum=w483, error in=w475) -> (error out=w484:errorcluster)  [unwired: 1 out]
            n181 = Build Array(w495) -> (w494:cluster{path[]}[])
          }
          frame 14 {
            # "Go through all supported AVI Codec options"
            n182 = for "This loop creates a new AVI for each compressor installed on your machine.\nThe new AVI copies images from an original uncompressed AVI.  While the frames are being copied,\nthe average write time is recorded.  When the AVI is finished writing, the file size is recorded and it is compared\nwith the original AVI to see how similar it is using a simple subtraction. \nThe average write time, file size, and quality are recorded in the Results table." {
              tunnel: w535 -> [w560]
              tunnel: w534 -> [w556] mode=indexing
              tunnel: [w544] -> w532 mode=indexing
              tunnel: [w548] -> w537 mode=indexing
              shift-right: [w547] -> w536
              shift-left: w533 -> [w559]
              tunnel: w531 -> [w543]
              shift-right: [w538] -> w529
              shift-left: w530 -> [w539]
              # "Create the AVI with the codec under test"
              n183 = Increment(x=w539) -> (x+1=w538:i32)
              n184 = Search and Replace String(replace all?=TRUE ("replace all? (F)"), input string=w556, search string=":" ("regular expression (\"\")")) -> (result string=w542:string)  [unwired: 5 in, 3 out]
              n185 = local write "Progress Bar"(w538) -> ()
              n186 = Format Into String(format string="AVI (%s)_0.avi", w542) -> (resulting string=w540:string)  [unwired: 2 in, 1 out]
              n187 = Build Path(base path=w560, name or relative path=w540) -> (appended path=w546:path)
              n188 = call "IMAQ AVI2 Create"("error in (no error)"=w559, "Codec"=w556, "AVI Path"=w546) -> ("error out"=w553:errorcluster, "AVI Refnum"=w558:T13)  [unwired: 2 in, 5 out]
              n189 = call "High Resolution Timer Helper.vi"("error in (no error)"=w553) -> ("error out"=w550:errorcluster, "Current Time"=w549:dbl)  [unwired: 8 in, 1 out]
              n190 = for {
                tunnel: w543 -> [w563] mode=indexing
                shift-right: [w562] -> w554
                shift-left: w558 -> [w564]
                shift-right: [w561] -> w552
                shift-left: w550 -> [w565]
                n191 = call "IMAQ AVI2 Write Frame"("error in (no error)"=w565, "Image"=w563, "AVI Refnum"=w564) -> ("error out"=w561:errorcluster, "AVI Refnum (duplicate)"=w562:T13)  [unwired: 7 out]
              }
              n192 = Build Array(w546) -> (w545:path[])
              n193 = Bundle(w545) -> (w544:cluster{path[]})  [unwired: 1 in]
              n194 = call "High Resolution Timer Helper.vi"("error in (no error)"=w552, "Previous Time"=w549) -> ("error out"=w551:errorcluster, "Time Difference (ms)"=w548:dbl)  [unwired: 7 in, 1 out]
              n195 = call "IMAQ AVI2 Close"("error in (no error)"=w551, "AVI Refnum"=w554) -> ("error out"=w547:errorcluster)  [unwired: 9 out]
            }
          }
        }
        n196 = Increment(x=w105) -> (x+1=w104:i32)
        "Progress Bar" <- w104
        n197 = Unbundle By Name(w103) -> ("status"=w108:bool)
        n198 = Boolean To (0,1)(Boolean=w108) -> (0, 1=w107:i16)
        n199 = Not(x=w108) -> (.not. x?=w109:bool)
        n200 = Add(x=w107, y=w104) -> (x+y=w106:i32)
      }
      n201 = Decrement(x=w44) -> (x-1=w43:i32)
      n202 = Array Size(array=w51) -> (size(s)=w50:i32)
      n203 = Add(x=w43, y=w50) -> (x+y=w49:i32)
      n204 = Multiply(x=w49, y=2) -> (x*y=w56:i32)
      n205 = Decrement(x=w56) -> (x-1=w39:i32)
      n206 = property on="Progress Bar" class="Slide (strict)"("Scale.Range:Maximum"=w39, "Data Entry Limits:Maximum"=w39) -> ()  [unwired: 2 in, 2 out]
      n207 = call "IMAQ Create"("Image Name"="Comparison Source", "Image Type"=w38) -> ("New Image"=w53:T3, "error out"=w40:errorcluster)  [unwired: 2 in, 1 out]
      n208 = Build Array (concatenate)(w35, w53) -> (w54:T3[])
      n209 = for {
        tunnel: w46 -> [w598] mode=indexing
        tunnel: w33 -> [w595] mode=indexing
        tunnel: w35 -> [w594]
        tunnel: w45 -> [w600]
        tunnel: w53 -> [w599]
        tunnel: w38 -> [w596]
        tunnel: [w587] -> w41 mode=indexing if=w566
        tunnel: w40 -> [w576]
        tunnel: w36 -> [w574]
        i -> [w602]
        w585 = "%.2f" ("format string")
        # "If all values are 1, report it's an exact match"
        # "Only add to table if no error"
        # "Invert the quality for sorting purposes so the lowest values are always the best (file size, write time and inverse Quality)"
        n210 = Unbundle(w598) -> (w593:path[])
        n211 = Add(x=w600, y=w602) -> (x+y=w601:i32)
        n212 = local write "Progress Bar"(w601) -> ()
        n213 = for {
          tunnel: [w607] -> w597 mode=indexing
          tunnel: [w608] -> w573 mode=concatenating
          tunnel: w594 -> [w611]
          tunnel: w599 -> [w620]
          shift-right: [w621] -> w588
          shift-left: w576 -> [w617]
          tunnel: w593 -> [w612] mode=indexing
          tunnel: w596 -> [w618]
          i -> [w610]
          # "Divide by the number of images to get file size per image"
          n214 = call <vilib>:"Get File Extension.vi"("error in (no error)"=w617, "file"=w612) -> ("error out"=w616:errorcluster, "lowercase file extension"=w619:string)  [unwired: 5 in, 3 out]
          n215 = File/Directory Info(path=w612) -> (size=w613:i64)  [unwired: 1 in, 6 out]
          n216 = case shown="\"bin\"" w619 {
            tunnel: [w625 w641 w663 w680] -> w608
            tunnel: [w629 w637 w659 w674] -> w621
            tunnel: w620 -> [w631 w636 w656 _]
            tunnel: w616 -> [w630 w635 w657 w682]
            tunnel: w612 -> [w632 w634 w658 w683]
            tunnel: w611 -> [w624 w633 w662 w681]
            tunnel: w618 -> [_ _ _ w677]
            tunnel: w610 -> [w623 _ _ _]
            frame Default {
              # "This is the case that handles formats that produce a single image file for each image. The other cases handle a single image file for multiple images"
              n217 = Index Array(array=w624, index=w623) -> (element=w622:T3)
              n218 = call "IMAQ ReadFile 2"("File Path"=w632, "error in (no error)"=w630, "Image"=w631) -> ("error out"=w628:errorcluster, "Image Out"=w627:T3)  [unwired: 4 in, 3 out]
              n219 = call "Calculate Image Quality.vi"("error in (no error)"=w628, "Image to Compare"=w627, "Expected Image"=w622) -> ("error out"=w629:errorcluster, "Quality"=w626:dbl)  [unwired: 7 in]
              n220 = Build Array(w626) -> (w625:dbl[])
            }
            frame "avi" {
              n221 = call "IMAQ AVI2 Open"("error in (no error)"=w635, "AVI File Path"=w634) -> ("error out"=w642:errorcluster, "AVI Refnum"=w639:T13)  [unwired: 8 in]
              n222 = for {
                tunnel: w633 -> [w643] mode=indexing
                tunnel: [w646] -> w641 mode=indexing
                shift-right: [w645] -> w640
                shift-left: w642 -> [w651]
                shift-right: [w649] -> w638
                shift-left: w639 -> [w652]
                tunnel: w636 -> [w648]
                i -> [w650]
                n223 = call "IMAQ AVI2 Read Frame"("error in (no error)"=w651, "Frame Number"=w650, "Image"=w648, "AVI Refnum"=w652) -> ("error out"=w647:errorcluster, "Image Out"=w644:T3, "AVI Refnum (duplicate)"=w649:T13)  [unwired: 5 in]
                n224 = call "Calculate Image Quality.vi"("error in (no error)"=w647, "Image to Compare"=w644, "Expected Image"=w643) -> ("error out"=w645:errorcluster, "Quality"=w646:dbl)  [unwired: 7 in]
              }
              n225 = call "IMAQ AVI2 Close"("error in (no error)"=w640, "AVI Refnum"=w638) -> ("error out"=w637:errorcluster)  [unwired: 9 out]
            }
            frame "tdms" {
              # "Use the asynchronous TDMS read since it is more efficient."
              n226 = call-poly "TDMS File Initialization (Poly).vi"("error in (no error)"=w657, "Image In"=w656, "File Path"=w658) -> ("error out"=w653:errorcluster, "Read Settings"=w654:T14, "TDMS Refnum Out"=w655:refnum<k34>)  [unwired: 5 in, 1 out]
              n227 = for {
                tunnel: w662 -> [w664] mode=indexing
                tunnel: [w673] -> w663 mode=indexing
                shift-right: [w672] -> w660
                shift-left: w653 -> [w669]
                shift-right: [w668] -> w661
                shift-left: w655 -> [w671]
                tunnel: w654 -> [w670]
                i -> [w665]
                n228 = call "TDMS Read File.vi"("error in"=w669, "Image Index"=w665, "Read Settings"=w670, "TDMS Refnum In"=w671) -> ("error out"=w667:errorcluster, "Image"=w666:T3, "TDMS Refnum Out"=w668:refnum<k34>)  [unwired: 4 in, 1 out]
                n229 = call "Calculate Image Quality.vi"("error in (no error)"=w667, "Image to Compare"=w666, "Expected Image"=w664) -> ("error out"=w672:errorcluster, "Quality"=w673:dbl)  [unwired: 7 in]
              }
              n230 = TDMS Advanced Close(8:w660, 11:w661) -> (0:w659:errorcluster)  [unwired: 2 in, 1 out]
            }
            frame "bin" {
              n231 = Open/Create/Replace File(file path (use dialog)=w683, error in=w682) -> (refnum out=w678:refnum<file>, error out=w679:errorcluster)  [unwired: 4 in, 1 out]
              n232 = for {
                tunnel: w681 -> [w685] mode=indexing
                tunnel: [w692] -> w680 mode=indexing
                shift-right: [w691] -> w676
                shift-left: w679 -> [w689]
                tunnel: w678 -> [w690]
                tunnel: w677 -> [w687]
                tunnel: [w686] -> w675
                n233 = case shown="0, Default" w687 {
                  tunnel: w690 -> [w698 w704 w710 w716]
                  tunnel: w689 -> [w697 w703 w709 w715]
                  tunnel: [w696 w702 w708 w714] -> w686
                  tunnel: [w694 w700 w706 w712] -> w688
                  tunnel: [w693 w699 w705 w711] -> w684
                  frame 0, Default {
                    n234 = Read from Binary File(5:u8[][] [], 8:w697, 11:w698) -> (0:w694:errorcluster, 2:w693:u8[][], 3:w696:refnum<file>)  [unwired: 3 in, 1 out]
                  }
                  frame 1 {
                    n235 = Read from Binary File(5:i16[][] [], 8:w703, 11:w704) -> (0:w700:errorcluster, 2:w699:i16[][], 3:w702:refnum<file>)  [unwired: 3 in, 1 out]
                  }
                  frame 4 {
                    n236 = Read from Binary File(5:u32[][] [], 8:w709, 11:w710) -> (0:w706:errorcluster, 2:w705:u32[][], 3:w708:refnum<file>)  [unwired: 3 in, 1 out]
                  }
                  frame 7 {
                    n237 = Read from Binary File(5:u16[][] [], 8:w715, 11:w716) -> (0:w712:errorcluster, 2:w711:u16[][], 3:w714:refnum<file>)  [unwired: 3 in, 1 out]
                  }
                }
                n238 = call "Calculate Image Quality.vi"("error in (no error)"=w688, "Image Pixels to Compare (U32)"=w684, "Expected Image"=w685) -> ("error out"=w691:errorcluster, "Quality"=w692:dbl)  [unwired: 7 in]
              }
              n239 = Close File(refnum=w675, error in=w676) -> (error out=w674:errorcluster)  [unwired: 1 out]
            }
          }
          n240 = To Double Precision Float(number=w613) -> (double precision float=w614:dbl)
          n241 = Divide(x=w614, y=1000.0) -> (x/y=w609:dbl)
          n242 = Array Size(array=w608) -> (size(s)=w606:i32)
          n243 = Max & Min(x=w606, y=1) -> (max(x,y)=w604:i32)  [unwired: 1 out]
          n244 = To Double Precision Float(number=w604) -> (double precision float=w603:dbl)
          n245 = Divide(x=w609, y=w603) -> (x/y=w607:dbl)
        }
        n246 = Index Array(array=w593) -> (element=w592:path)  [unwired: 1 in]
        n247 = Strip Path(path=w592) -> (name=w591:string)  [unwired: 1 out]
        n248 = Divide(x=w595, y=w574) -> (x/y=w578:dbl)
        n249 = Match Pattern(string=w591, regular expression="_") -> (before substring=w579:string)  [unwired: 1 in, 3 out]
        n250 = Equal?(x=1.0, y=w573) -> (x = y?=w571:bool[])
        n251 = Unbundle By Name(w588) -> ("status"=w589:bool)
        n252 = call-poly <vilib>:"Mean.vi"("X"=w597) -> ("mean"=w577:dbl)  [unwired: 1 out]
        n253 = call-poly <vilib>:"Mean.vi"("X"=w573) -> ("mean"=w575:dbl)  [unwired: 1 out]
        n254 = And Array Elements(Boolean array=w571) -> (logical AND=w570:bool)
        n255 = Format Into String(format string=w585, w578) -> (resulting string=w580:string)  [unwired: 2 in, 1 out]
        n256 = Format Into String(format string=w585, w577) -> (resulting string=w582:string)  [unwired: 2 in, 1 out]
        n257 = Subtract(x=1.0, y=w575) -> (x-y=w584:dbl)
        n258 = Select(t="Yes", s=w570, f="No") -> (s? t:f=w568:string)
        n259 = Not(x=w589) -> (.not. x?=w566:bool)
        n260 = Build Array(w579, w580, w582, w568) -> (w581:string[])
        n261 = Bundle(cluster=T9 {"Table Data"=[], "Description"="", "Write time"=0.0, "File Size"=0.0, "Sort Quality"=0.0} ("output cluster"), "Table Data"=w581, "Description"=w579, "Write time"=w578, "File Size"=w577, "Sort Quality"=w584) -> (w587:T9)
      }
      n262 = while {
        tunnel: w41 -> [w65]
        stop <- "Stop" stop-if-true
        n263 = feedback #1() -> (w63:bool)  [unwired: 1 in]
        n264 = feedback-in #1("Show Only Lossless") -> ()
        n265 = feedback-in #2("Sort By") -> ()
        n266 = feedback #2(enum16{"Write Time", "File Size"}."Write Time" ("Sort By")) -> (w71:enum16{"Write Time", "File Size"})
        n267 = First Call?() -> (First Call?: T/F=w69:bool)
        n268 = Not Equal?(x="Show Only Lossless", y=w63) -> (x != y?=w62:bool)
        n269 = Not Equal?(x="Sort By", y=w71) -> (x != y?=w70:bool)
        n270 = Compound Arithmetic op=OR(w69, w70, w62) -> (w68:bool)
        n271 = case shown="True" w68 {
          tunnel: "Sort By" -> [_ w76]
          tunnel: w65 -> [_ w77]
          tunnel: "Show Only Lossless" -> [_ w74]
          frame False {
            n272 = Wait (ms)(milliseconds to wait=u32 100) -> ()  [unwired: 1 out]
          }
          frame True {
            # "When Sort Quality is 0, that means images exactly match."
            n273 = case shown="\"Write Time\"" w76 {
              tunnel: w77 -> [w87 w95]
              tunnel: [w85 w93] -> w75
              frame "Write Time" {
                n274 = for {
                  tunnel: w87 -> [w90] mode=indexing
                  tunnel: [w89] -> w86 mode=indexing
                  n275 = Unbundle By Name(w90) -> ("Write time"=w92:dbl, "Sort Quality"=w91:dbl, "Table Data"=w88:string[])
                  n276 = Bundle("Write time"=w92, "Sort Quality"=w91, "Table Data"=w88) -> (w89:T15)  [unwired: 1 in]
                }
                n277 = Sort 1D Array(array=w86) -> (sorted array=w85:T16)
              }
              frame "File Size" {
                n278 = for {
                  tunnel: w95 -> [w98] mode=indexing
                  tunnel: [w97] -> w94 mode=indexing
                  n279 = Unbundle By Name(w98) -> ("File Size"=w100:dbl, "Sort Quality"=w99:dbl, "Table Data"=w96:string[])
                  n280 = Bundle("File Size"=w100, "Sort Quality"=w99, "Table Data"=w96) -> (w97:T17)  [unwired: 1 in]
                }
                n281 = Sort 1D Array(array=w94) -> (sorted array=w93:T18)
              }
            }
            n282 = for {
              tunnel: w75 -> [w84] mode=indexing
              tunnel: [w83] -> w73 mode=indexing if=w78
              tunnel: w74 -> [w81]
              w79 = TRUE  # Show All
              n283 = Unbundle By Name(w84) -> ("Table Data"=w83:string[], "Sort Quality"=w82:dbl)
              n284 = Equal To 0?(x=w82) -> (x = 0?=w80:bool)
              n285 = Select(t=w80, s=w81, f=w79) -> (s? t:f=w78:bool)
            }
            n286 = property on="Results" class="MCListbox (strict)"("Item Names"=w73) -> ()  [unwired: 2 in, 2 out]
          }
        }
      }
      n287 = flat-sequence {
        tunnel: w41 -> [_]
        frame #0 {
          w59 = T2."Enabled" ("Disabled")
          # "Now that benchmarking is complete, enable the Sort By and Stop controls."
          n288 = property on="Progress Bar" class="Slide (strict)"() -> ("Data Entry Limits:Maximum"=w60:dbl)  [unwired: 2 in, 2 out]
          n289 = property on="Sort By" class="Enum (strict)"("DisabledEnum"=w59) -> ()  [unwired: 2 in, 2 out]
          n290 = local write "Progress Bar"(w60) -> ()
          n291 = property on="Stop" class="Bool"("DisabledEnum"=w59) -> ()  [unwired: 2 in, 2 out]
          n292 = property on="Show Only Lossless" class="Bool (strict)"("DisabledEnum"=w59) -> ()  [unwired: 2 in, 2 out]
        }
      }
      "Results" <- -1 ("Results")
    }
    frame Error {
      # "Ignore any errors in the other case and just don't include any file formats that don't work in the resulting table."
      n293 = call <vilib>:"Simple Error Handler.vi"("error in (no error)"=w718) -> ()  [unwired: 1 in, 8 out]
    }
  }
  n294 = for {
    tunnel: w26 -> [w719] mode=indexing
    n295 = call "IMAQ Dispose"("Image"=w719) -> ()  [unwired: 2 in, 4 out]
  }
